vi "RpR.vi"(0 "R2":dbl, 1 "R1":dbl) -> (2 "R1 + R2":dbl, 3 "R1 // R2":dbl, 4 "R1 * R2":dbl)   [LabVIEW 2010]
doc: "Calculate parallel resistance of two passive circuit elements\n\nR1 // R2 = ( ( R1 * R2 ) / ( R1 + R2 ) )"
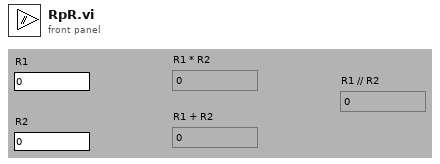
[diagram p1: front panel]
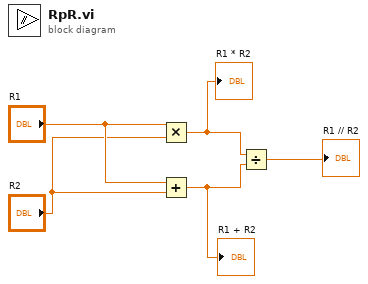
[diagram p0: block diagram]
diagram:
  n1 = Multiply(x="R1", y="R2") -> (x*y=w2:dbl)
  "R1 * R2" <- w2
  n2 = Add(x="R1", y="R2") -> (x+y=w1:dbl)
  "R1 + R2" <- w1
  n3 = Divide(x=w2, y=w1) -> (x/y=→"R1 // R2":dbl)
